vi "U01_8_2 OpenExcelActiveX.vi"(8 "error in":errorcluster) -> (0 "error out":errorcluster, 2 "IsOpened?":bool, 3 "Reference":T1)   [LabVIEW 2019]
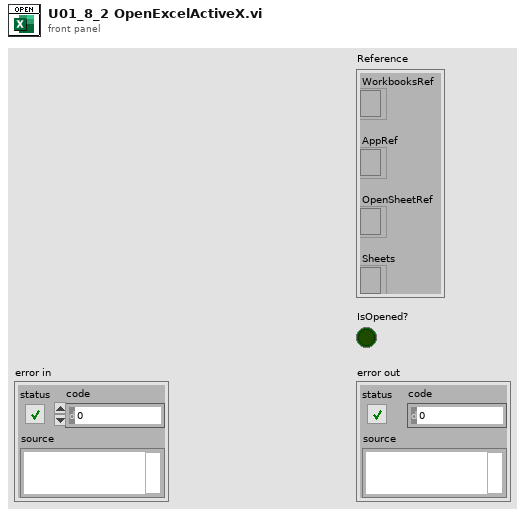
[diagram p1: front panel]
types:
  T1 = cluster{"AppRef":refnum<k7>, "WorkbooksRef":refnum<k7>, "OpenSheetRef":refnum<k7>, "Sheets":refnum<k7>}
  T2 = cluster{"Excel._Application":refnum<k7>, "Workbooks":refnum<k7>, "Open":refnum<k7>, "Sheets":refnum<k7>}
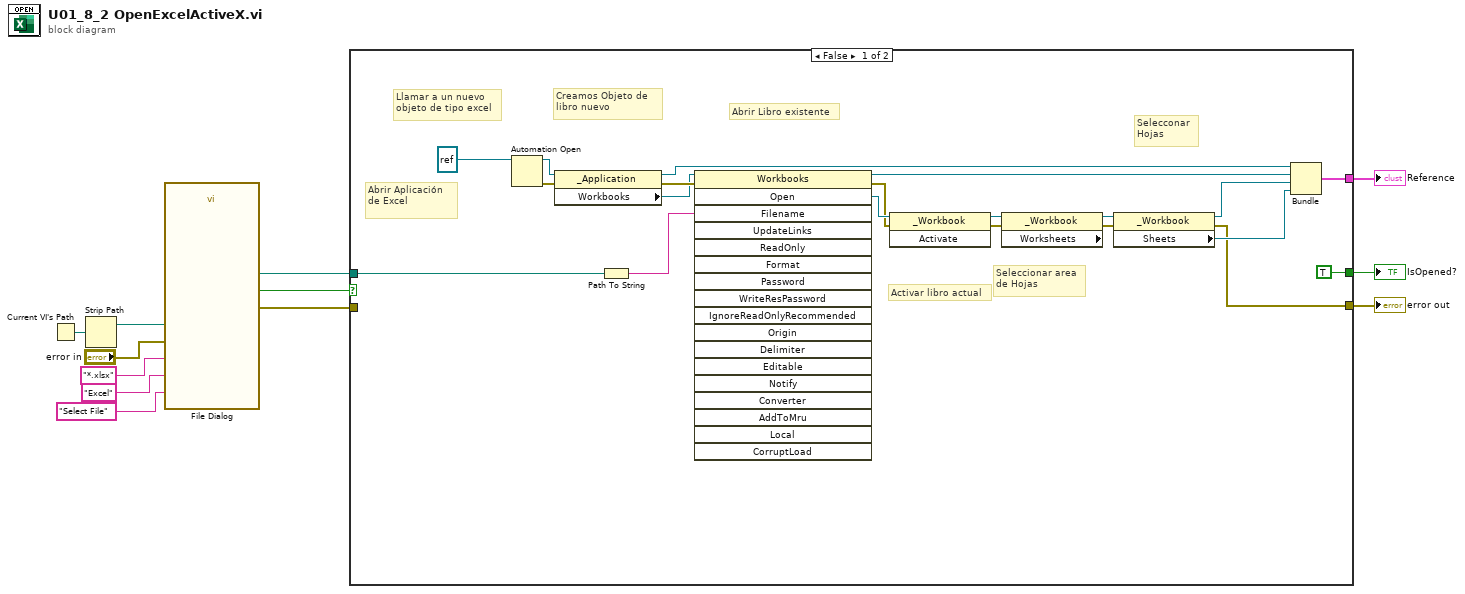
[diagram p0: block diagram]
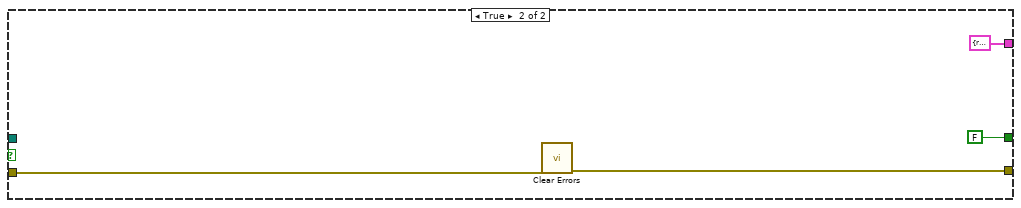
[diagram p2: hidden frame]
diagram:
  n1 = Current VI's Path() -> (path=w9:path)
  n2 = Strip Path(path=w9) -> (stripped path=w5:path)  [unwired: 1 out]
  n3 = call "File Dialog"("start path"=w5, "prompt"="Select File", "error in"="error in", "pattern (all files)"="*.xlsx", "pattern label"="Excel") -> ("selected path"=w12:path, "cancelled"=w11:bool, "error out"=w10:errorcluster)  [unwired: 7 in, 1 out]
  n4 = case shown="False" w11 {
    tunnel: w12 -> [w15 _]
    tunnel: w10 -> [_ w36]
    tunnel: [TRUE FALSE] -> w3
    tunnel: [w16 T2 {"Excel._Application"=refnum, "Workbooks"=refnum, "Open"=refnum, "Sheets"=refnum}] -> w2
    tunnel: [w14 w34] -> w1
    frame False {
      # "Selecconar \nHojas"
      # "Seleccionar area \nde Hojas"
      # "Activar libro actual"
      # "Abrir Libro existente"
      # "Creamos Objeto de \nlibro nuevo"
      # "Llamar a un nuevo \nobjeto de tipo excel"
      # "Abrir Aplicación \nde Excel"
      n5 = Automation Open(Automation Refnum=refnum<k7> refnum ("Excel._Application")) -> (Automation Refnum=w22:refnum<k7>, error out=w23:errorcluster)  [unwired: 3 in]
      n6 = property class="_Application"(reference=w22, error in=w23) -> (reference out=w17:refnum<k7>, error out=w25:errorcluster, "Workbooks"=w24:refnum<k7>)
      n7 = Path To String(path=w15) -> (string=w32:string)
      n8 = invoke class="Workbooks" method="Open"(reference=w24, error in=w25, "Filename"=w32) -> (reference out=w18:refnum<k7>, error out=w26:errorcluster, "Open"=w31:refnum<k7>)  [unwired: 15 in, 15 out]
      n9 = invoke class="_Workbook" method="Activate"(reference=w31, error in=w26) -> (reference out=w27:refnum<k7>, error out=w28:errorcluster)  [unwired: 1 in, 1 out]
      n10 = property class="_Workbook" props=["Worksheets"](reference=w27, error in=w28) -> (reference out=w29:refnum<k7>, error out=w30:errorcluster)  [unwired: 1 out]
      n11 = property class="_Workbook"(reference=w29, error in=w30) -> (reference out=w19:refnum<k7>, error out=w14:errorcluster, "Sheets"=w20:refnum<k7>)
      n12 = Bundle("Excel._Application"=w17, "Workbooks"=w18, "Open"=w19, "Sheets"=w20) -> (w16:T2)  [unwired: 1 in]
    }
    frame True {
      n13 = call <vilib>:"Clear Errors.vi"("error in (no error)"=w36) -> ("error out"=w34:errorcluster)  [unwired: 5 in, 1 out]
    }
  }
  "IsOpened?" <- w3
  "Reference" <- w2
  "error out" <- w1
